vi "QuadraticDiscriminantAnalysis.vi"(8 "error in":errorcluster) -> (0 "error out":errorcluster, 3 "out":refnum<class "QuadraticDiscriminantAnalysis.lvclass">)   [LabVIEW 2020]
doc: "Quadratic Discriminant Analysis\n\n A classifier with a quadratic decision boundary, generated\n by fitting class conditional densities to the data\n and using Bayes' rule.\n\n The model fits a Gaussian density to each class.\n\n .. versionadded:: 0.17\n *QuadraticDiscriminantAnalysis*\n\n Read more in the :ref:`User Guide <lda_qda>`.\n\n Parameters\n ----------\n priors : ndarray of shape (n_classes,), default=None\n Class priors. By default, the class proportions are inferred from the\n training data.\n\n reg_param : float, default=0.0\n Regularizes the per-class covariance estimates by transforming S2 as\n ``S2 = (1 - reg_param) * S2 + reg_param * np.eye(n_features)``,\n where S2 corresponds to the `scaling_` attribute of a given class.\n\n store_covariance : bool, default=False\n If True, the class covariance matrices are explicitely computed and\n stored in the `self.covariance_` attribute.\n\n .. versionadded:: 0.17\n\n tol : float, default=1.0e-4\n Absolute threshold for a singular value to be considered significant,\n used to estimate the rank of `Xk` where `Xk` is the centered matrix\n of samples in class k. This parameter does not affect the\n predictions. It only controls a warning that is raised when features\n are considered to be colinear.\n\n .. versionadded:: 0.17\n\n Attributes\n ----------\n covariance_ : list of len n_classes of ndarray of shape (n_features, n_features)\n For each class, gives the covariance matrix estimated using the\n samples of that class. The estimations are unbiased. Only present if\n `store_covariance` is True.\n\n means_ : array-like of shape (n_classes, n_features)\n Class-wise means.\n\n priors_ : array-like of shape (n_classes,)\n Class priors (sum to 1).\n\n rotations_ : list of len n_classes of ndarray of shape (n_features, n_k)\n For each class k an array of shape (n_features, n_k), where\n ``n_k = min(n_features, number of elements in class k)``\n It is the rotation of the Gaussian distribution, i.e. its\n principal axis. It corresponds to `V`, the matrix of eigenvectors\n coming from the SVD of `Xk = U S Vt` where `Xk` is the centered\n matrix of samples from class k.\n\n scalings_ : list of len n_classes of ndarray of shape (n_k,)\n For each class, contains the scaling of\n the Gaussian distributions along its principal axes, i.e. the\n variance in the rotated coordinate system. It corresponds to `S^2 /\n (n_samples - 1)`, where `S` is the diagonal matrix of singular values\n from the SVD of `Xk`, where `Xk` is the centered matrix of samples\n from class k.\n\n classes_ : ndarray of shape (n_classes,)\n Unique class labels.\n\n \nAvailable methods:\nDecision Function\nFit\nPredict\nPredict Log Proba\nPredict Proba\nScore\nGet Attributes\nGet Params\nSet Params"
uses:
  QuadraticDiscriminantAnalysis.lvclass
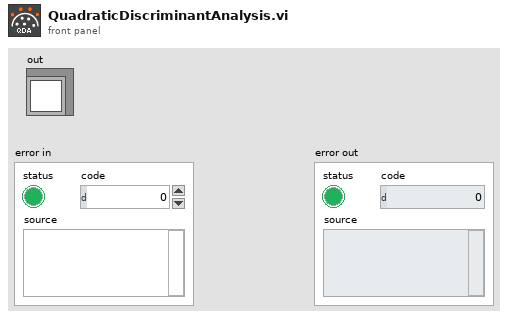
[diagram p1: front panel]
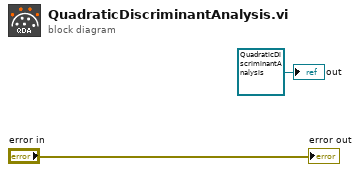
[diagram p0: block diagram]
diagram:
  "out" <- refnum<class "QuadraticDiscriminantAnalysis.lvclass"> refnum ("model")
  "error out" <- "error in"
